vi "Motor Control.vi"() -> ()   [LabVIEW 2020]
uses:
  <vilib>/MakerHub/LINX/Public/Peripherals/PWM/PWM Set Duty Cycle 1 Chan.vi
  <vilib>/MakerHub/LINX/Public/Peripherals/Digital/Digital Write N Chans.vi
  <vilib>/MakerHub/LINX/Private/Local IO/LinxDigitalWrite.vi
  <vilib>/MakerHub/LINX/Public/Utilities/Check Channel.vi
  <vilib>/MakerHub/LINX/Public/Utilities/Open Serial.vi
  <vilib>/MakerHub/LINX/Public/Peripherals/PWM/PWM Set Duty Cycle N Chans.vi
  <vilib>/MakerHub/LINX/Private/Utilties/Generate Error.vi
  <vilib>/MakerHub/LINX/LMH-LINX.lvlib
panel:
  in  "STOP":bool
  in  "Motor Direction":bool[](array[boolean])
  in  "Duty Cycle (0-1)":dbl(slide) min=0.0 max=1.0 step=0.0005 scale=0.0..1.0
  in  "Serial Port":refnum<visa-resource-name>="N/A"
  # "PIN 7"
  # "PIN 8"
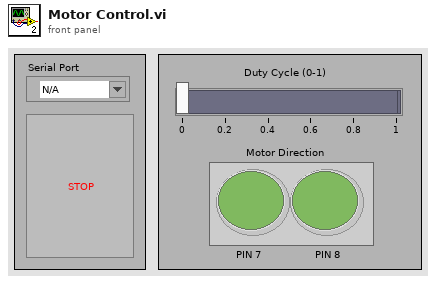
[diagram p1: front panel]
types:
  T1 = typedef "LMH-LINX.lvlib/LINX Ref.ctl" = cluster{"IO":T2, "Interface":T3, "LINX Device Config":T4}
  T2 = typedef "LMH-LINX.lvlib/Platform.ctl" = enum16{"Remote", "Local"}
  T3 = typedef "LMH-LINX.lvlib/Interface.ctl" = enum16{"Serial", "TCP"}
  T4 = typedef "LMH-LINX.lvlib/Device.lvlib/LINX Device Config.ctl" = cluster{"Interface":T3, "COM Port":refnum<visa-resource-name>, "TCP Configuration":T5, "Device Family":u8, "Device ID":u8, "Device Name":string, "TCP Ref":refnum<k5>, "Channels":T6}
  T5 = typedef "LMH-LINX.lvlib/Device.lvlib/TCP Config.ctl" = cluster{"IP Address":string, "Port":u16}
  T6 = typedef "LMH-LINX.lvlib/Channels.ctl" = cluster{"DI":u8[], "DO":u8[], "AI":u8[], "AO":u8[], "PWM":u8[], "QE":u8[], "UART":u8[], "I2C 2":u8[], "SPI":u8[], "CAN":u8[], "Servo":u8[], "AI Ref (V)":dbl, "AI Resolution (Bits)":u8, "AO Ref (V)":dbl, "AO Resolution (Bits)":u8}
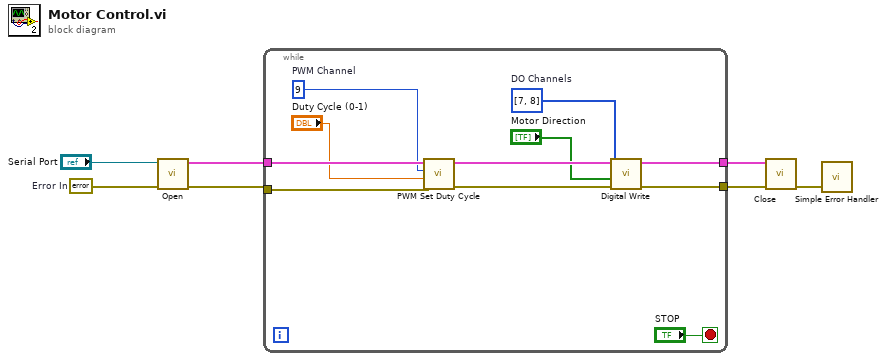
[diagram p0: block diagram]
diagram:
  w4 = errorcluster {"status"=FALSE, "code"=0, "source"=""}  # Error In
  n1 = call-poly <vilib>:"Open.vi"("Error In"=w4, "Serial Port"="Serial Port") -> ("Error Out"=w6:errorcluster, "LINX Resource"=w7:T1)  [unwired: 7 in, 1 out]
  n2 = while {
    tunnel: w7 -> [w18]
    tunnel: w6 -> [w17]
    tunnel: [w12] -> w2
    tunnel: [w11] -> w3
    stop <- "STOP" stop-if-true
    w16 = u8 9  # PWM Channel
    w8 = u8[] [7, 8]  # DO Channels
    n3 = call-poly <vilib>:"PWM Set Duty Cycle.vi"("Error In"=w17, "Duty Cycle (0-1)"="Duty Cycle (0-1)", "PWM Channel"=w16, "LINX Resource"=w18) -> ("Error Out"=w13:errorcluster, "LINX Resource"=w14:T1)  [unwired: 6 in]
    n4 = call-poly <vilib>:"Digital Write.vi"("Error In"=w13, "Values"="Motor Direction", "DO Channels"=w8, "LINX Resource"=w14) -> ("Error Out"=w12:errorcluster, "LINX Resource"=w11:T1)  [unwired: 6 in]
  }
  n5 = call <vilib>:"Close.vi"("Error In"=w2, "LINX Resource"=w3) -> ("Error Out"=w1:errorcluster)  [unwired: 9 in]
  n6 = call <vilib>:"Simple Error Handler.vi"("error in (no error)"=w1) -> ()  [unwired: 4 in, 5 out]
